vi "Input Impedence_Time Domain(SubVI).vi"(10 "Ad (m^2)":dbl, 11 "PWV (m/s)":dbl) -> (3 "Zc (mmHg/ml/s)":dbl=18.84214783526999)   [LabVIEW 2017]
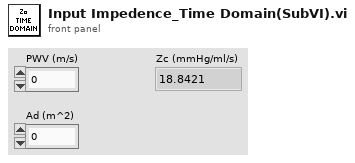
[diagram p1: front panel]
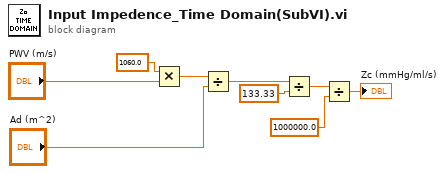
[diagram p0: block diagram]
diagram:
  n1 = Multiply(x=1060.0, y="PWV (m/s)") -> (x*y=w2:dbl)
  n2 = Divide(x=w2, y="Ad (m^2)") -> (x/y=w4:dbl)
  n3 = Divide(x=w4, y=133.33) -> (x/y=w6:dbl)
  n4 = Divide(x=w6, y=1000000.0) -> (x/y=→"Zc (mmHg/ml/s)":dbl)
